vi "FRCts_ClientAPI_Error Handler.vi"(8 "error in (no error)":errorcluster, 9 "HTTP Response":string, 10 "4xx Warning?":bool, 11 "HTTP Code":i32) -> (0 "error out":errorcluster)   [LabVIEW 2014, in "FRCts_ClientAPI.lvlib"]
doc: "This VI handles errors returned from HTTP actions."
uses:
  FRCts_ClientAPI.lvlib
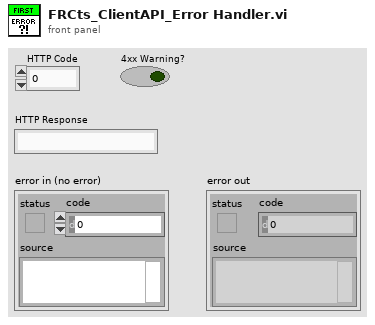
[diagram p1: front panel]
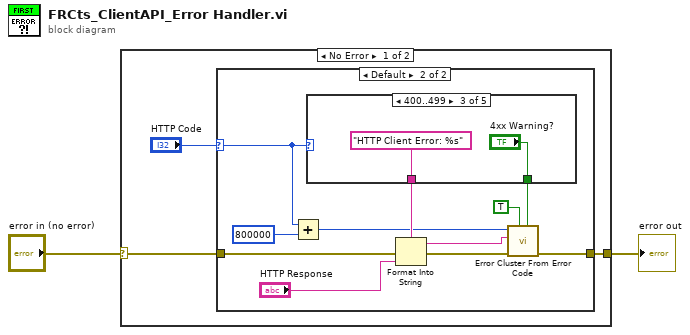
[diagram p0: block diagram]
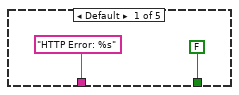
[diagram p3: hidden frame]
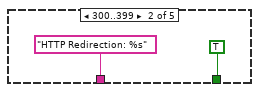
[diagram p4: hidden frame]
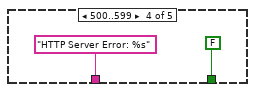
[diagram p5: hidden frame]
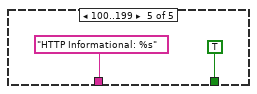
[diagram p6: hidden frame]
diagram:
  n1 = case shown="No Error" "error in (no error)" {
    selector: "error in (no error)" -> [w5 w28]
    tunnel: [w4 w28] -> w1
    frame No Error {
      n2 = case shown="Default" "HTTP Code" {
        selector: "HTTP Code" -> [_ w7]
        tunnel: w5 -> [w6 w16]
        tunnel: [w6 w8] -> w4
        frame 200..299 {
        }
        frame Default {
          n3 = Add(x=w7, y=800000) -> (x+y=w9:i32)
          n4 = case shown="400..499" w7 {
            tunnel: ["HTTP Error: %s" ("format string") "HTTP Redirection: %s" ("format string") "HTTP Client Error: %s" ("format string") "HTTP Server Error: %s" ("format string") "HTTP Informational: %s" ("format string")] -> w14
            tunnel: [FALSE ("is warning? (False)") TRUE ("is warning? (False)") "4xx Warning?" FALSE ("is warning? (False)") TRUE ("is warning? (False)")] -> w12
            frame Default {
            }
            frame 300..399 {
            }
            frame 400..499 {
            }
            frame 500..599 {
            }
            frame 100..199 {
            }
          }
          n5 = Format Into String(format string=w14, error in=w16, "HTTP Response") -> (resulting string=w10:string, error out=w13:errorcluster)  [unwired: 1 in]
          n6 = call <vilib>:"Error Cluster From Error Code.vi"("is warning? (False)"=w12, "show call chain? (False)"=TRUE, "error in (no error)"=w13, "error message (\"\")"=w10, "error code (0)"=w9) -> ("error out"=w8:errorcluster)  [unwired: 4 in]
        }
      }
    }
    frame Error {
    }
  }
  "error out" <- w1
